vi "get_context.vi"(8 "error in (no error)":errorcluster, 11 "WebSocket Logger in":refnum<class "WebSocket Logger.lvclass">) -> (0 "error out":errorcluster, 1 "remote address":string, 2 "remote port":u16, 3 "WebSocket Logger out":refnum<class "WebSocket Logger.lvclass">)   [LabVIEW 2019, in "WebSocket Server Toolkit.lvlib" / "WebSocket Logger.lvclass"]
uses:
  WebSocket Logger.lvclass
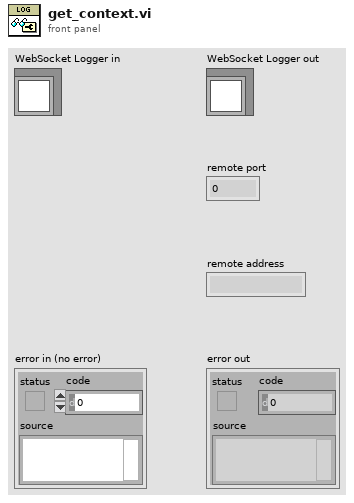
[diagram p1: front panel]
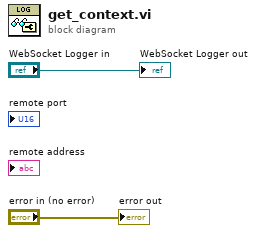
[diagram p0: block diagram]
diagram:
  "error out" <- "error in (no error)"
  "WebSocket Logger out" <- "WebSocket Logger in"
